vi "Write DeviceName.vi"(8 "error in (no error)":errorcluster, 10 "DeviceName":string, 11 "SCD in":refnum<class "SCD.lvclass">) -> (0 "error out":errorcluster, 3 "SCD out":refnum<class "SCD.lvclass">)   [LabVIEW 2023, in "SCD.lvclass"]
uses:
  SCD.lvclass
  GenericDevice/GenericDevice.lvclass
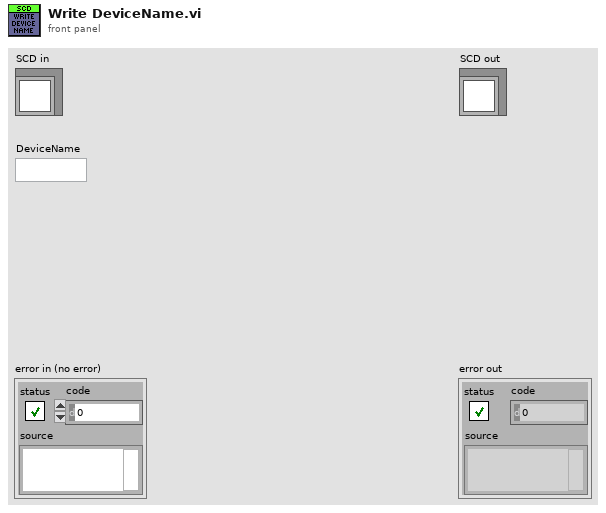
[diagram p1: front panel]
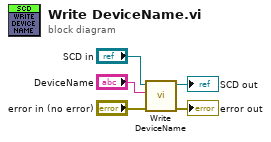
[diagram p0: block diagram]
diagram:
  n1 = call-parent "Write DeviceName.vi"("error in (no error)"="error in (no error)", "DeviceName"="DeviceName", "GenericDevice in"="SCD in") -> ("error out"=→"error out":errorcluster, "GenericDevice out"=→"SCD out":refnum<class "SCD.lvclass">)  [unwired: 7 in]
